vi "Close Session.vi"(8 "error in (no error)":errorcluster, 11 "MB_Serial session":refnum<class "MB_Master_Serial.lvclass">) -> (0 "error out":errorcluster)   [LabVIEW 2012, in "MB Master.lvlib" / "MB_Master_Serial.lvclass"]
doc: "Close the Modbus session. This will release the mutex and close the serial port."
uses:
  MB_Master_Serial.lvclass
  MB_Master_Serial.lvclass/MB_Master_Serial.ctl
  MB_VISA_Lock/MB_VISA_Lock.lvlib
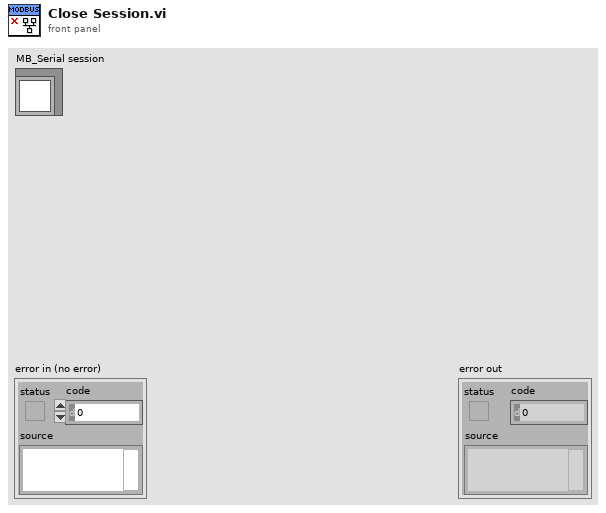
[diagram p1: front panel]
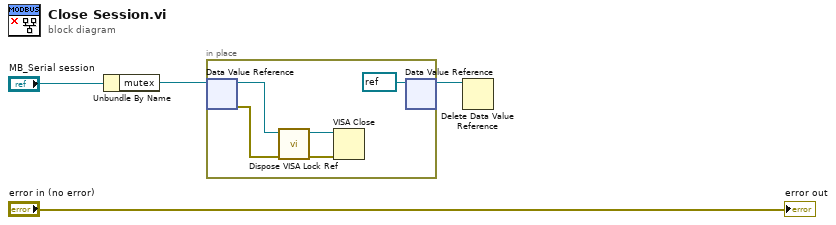
[diagram p0: block diagram]
diagram:
  n1 = Unbundle By Name("MB_Serial session") -> ("mutex"=w2:refnum<data-value>)
  n2 = in-place {
    n3 = in-place-dvr #1(w2) -> (w8:refnum<visa-resource-name>, w5:errorcluster)
    n4 = call "Dispose VISA Lock Ref.vi"("error in (no error)"=w5, "VISA session in"=w8) -> ("error out"=w9:errorcluster, "VISA session out"=w7:refnum<visa-resource-name>)  [unwired: 8 in]
    n5 = VISA Close(VISA resource name=w7, error in (no error)=w9) -> ()  [unwired: 1 out]
    n6 = in-place-dvr #1(refnum<visa-resource-name> refnum ("data value")) -> (w1:refnum<data-value>)  [unwired: 1 out]
  }
  n7 = Delete Data Value Reference(data value reference=w1) -> ()  [unwired: 1 in, 2 out]
  "error out" <- "error in (no error)"
